vi "Reset.vi"(8 "error in (no error)":errorcluster, 11 "Request in":refnum<class "Request.lvclass">) -> (0 "error out":errorcluster, 3 "Request out":refnum<class "Request.lvclass">)   [LabVIEW 2020, in "HTTP Utils.lvlib" / "Request.lvclass"]
doc: "Resets the internal state of the request without closing the connection. This is used to enable reusing established connections (and TLS handshaking) across multiple requests when the Connection: keep-alive header value is set.\n\nCalling this VI ensures any temporary file uploads from the previous request are deleted and only reuses the underlying client connection."
uses:
  Request.lvclass
  Request.lvclass/Request.ctl
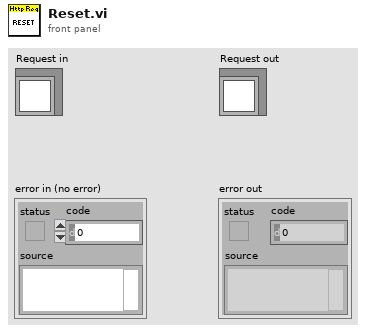
[diagram p1: front panel]
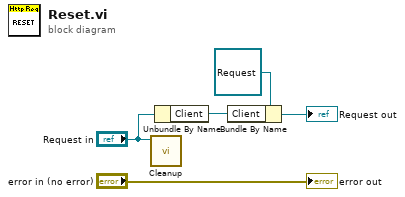
[diagram p0: block diagram]
diagram:
  n1 = call "Cleanup.vi"("Request in"="Request in") -> ()  [unwired: 10 in, 1 out]
  n2 = Unbundle By Name("Request in") -> ("Client"=w1:refnum<class "URI.lvclass">)
  n3 = Bundle By Name(cluster=refnum<class "Request.lvclass"> refnum ("Request out"), "Client"=w1) -> (→"Request out":refnum<class "Request.lvclass">)
  "error out" <- "error in (no error)"
